vi "1553B_帧解析_字符串_v4.vi"(11 "输入簇":T1) -> (2 "脉冲数":string, 3 "温度":string)   [LabVIEW 2012]
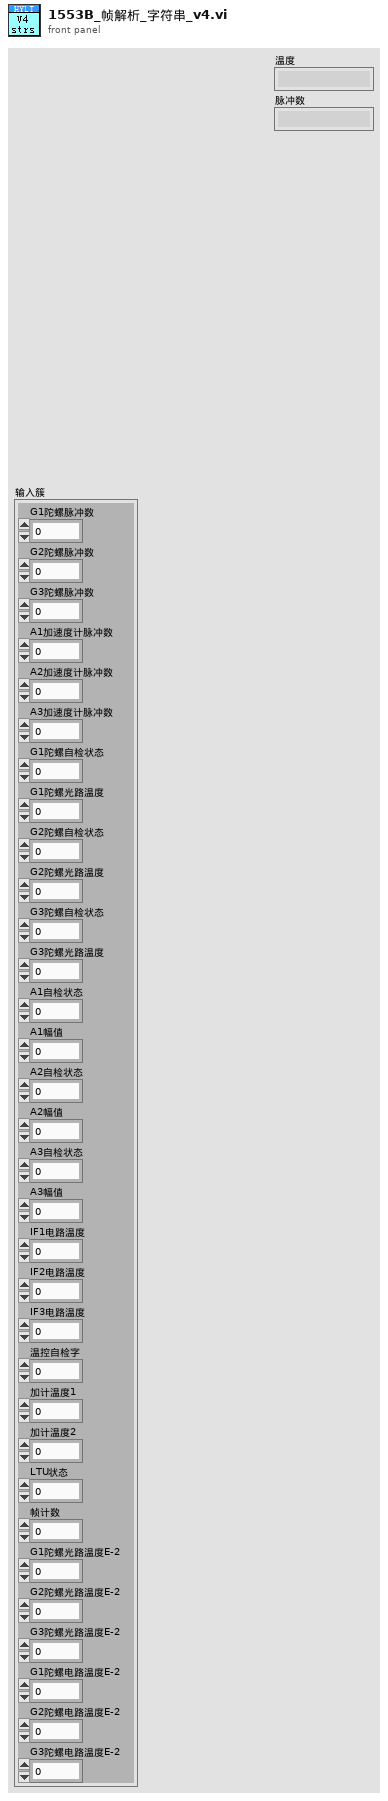
[diagram p1: front panel]
types:
  T1 = cluster{"G1陀螺脉冲数":i32, "G2陀螺脉冲数":i32, "G3陀螺脉冲数":i32, "A1加速度计脉冲数":i16, "A2加速度计脉冲数":i16, "A3加速度计脉冲数":i16, "G1陀螺自检状态":u8, "G1陀螺光路温度":i8, "G2陀螺自检状态":u8, "G2陀螺光路温度":i8, "G3陀螺自检状态":u8, "G3陀螺光路温度":i8, "A1自检状态":u8, "A1幅值":u8, "A2自检状态":u8, "A2幅值":u8, "A3自检状态":u8, "A3幅值":u8, "IF1电路温度":i8, "IF2电路温度":i8, "IF3电路温度":i8, "温控自检字":u8, "加计温度1":i16, "加计温度2":i16, "LTU状态":u8, "帧计数":u8, "G1陀螺光路温度E-2":i16, "G2陀螺光路温度E-2":i16, "G3陀螺光路温度E-2":i16, "G1陀螺电路温度E-2":i16, "G2陀螺电路温度E-2":i16, "G3陀螺电路温度E-2":i16}
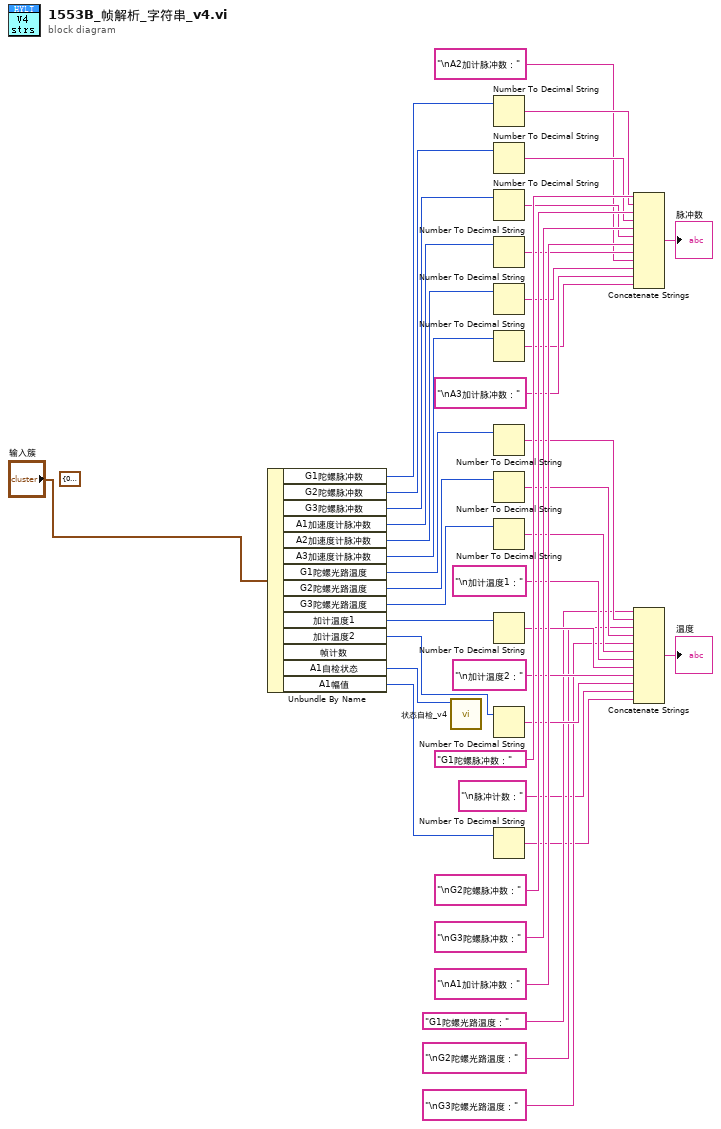
[diagram p0: block diagram]
diagram:
  (unwired) T1 {"G1陀螺脉冲数"=0, "G2陀螺脉冲数"=0, "G3陀螺脉冲数"=0, "A1加速度计脉冲数"=0, "A2加速度计脉冲数"=0, "A3加速度计脉冲数"=0, "G1陀螺自检状态"=0, "G1陀螺光路温度"=0, "G2陀螺自检状态"=0, "G2陀螺光路温度"=0, "G3陀螺自检状态"=0, "G3陀螺光路温度"=0, "A1自检状态"=0, "A1幅值"=0, "A2自检状态"=0, "A2幅值"=0, "A3自检状态"=0, "A3幅值"=0, "IF1电路温度"=0, "IF2电路温度"=0, "IF3电路温度"=0, "温控自检字"=0, "加计温度1"=0, "加计温度2"=0, "LTU状态"=0, "帧计数"=0, "G1陀螺光路温度E-2"=0, "G2陀螺光路温度E-2"=0, "G3陀螺光路温度E-2"=0, "G1陀螺电路温度E-2"=0, "G2陀螺电路温度E-2"=0, "G3陀螺电路温度E-2"=0} ("输入簇")
  n1 = Unbundle By Name("输入簇") -> ("G1陀螺脉冲数"=w25:i32, "G2陀螺脉冲数"=w24:i32, "G3陀螺脉冲数"=w23:i32, "A1加速度计脉冲数"=w22:i16, "A2加速度计脉冲数"=w39:i16, "A3加速度计脉冲数"=w38:i16, "G1陀螺光路温度"=w11:i8, "G2陀螺光路温度"=w10:i8, "G3陀螺光路温度"=w9:i8, "加计温度1"=w8:i16, "加计温度2"=w7:i16, "A1自检状态"=w40:u8, "A1幅值"=w3:u8)  [unwired: 1 out]
  n2 = call "状态自检_v4.vi"("陀螺自检状态字"=w40) -> ()  [unwired: 10 in, 1 out]
  n3 = Number To Decimal String(number=w25) -> (decimal integer string=w36:string)  [unwired: 1 in]
  n4 = Number To Decimal String(number=w24) -> (decimal integer string=w34:string)  [unwired: 1 in]
  n5 = Number To Decimal String(number=w23) -> (decimal integer string=w32:string)  [unwired: 1 in]
  n6 = Number To Decimal String(number=w22) -> (decimal integer string=w30:string)  [unwired: 1 in]
  n7 = Number To Decimal String(number=w39) -> (decimal integer string=w28:string)  [unwired: 1 in]
  n8 = Number To Decimal String(number=w38) -> (decimal integer string=w26:string)  [unwired: 1 in]
  n9 = Number To Decimal String(number=w11) -> (decimal integer string=w13:string)  [unwired: 1 in]
  n10 = Number To Decimal String(number=w10) -> (decimal integer string=w15:string)  [unwired: 1 in]
  n11 = Number To Decimal String(number=w9) -> (decimal integer string=w17:string)  [unwired: 1 in]
  n12 = Number To Decimal String(number=w8) -> (decimal integer string=w19:string)  [unwired: 1 in]
  n13 = Number To Decimal String(number=w7) -> (decimal integer string=w21:string)  [unwired: 1 in]
  n14 = Number To Decimal String(number=w3) -> (decimal integer string=w2:string)  [unwired: 1 in]
  n15 = Concatenate Strings("G1陀螺脉冲数：" ("字符串"), w36, "\nG2陀螺脉冲数：" ("字符串"), w34, "\nG3陀螺脉冲数：" ("字符串"), w32, "\nA1加计脉冲数：" ("字符串"), w30, "\nA2加计脉冲数：" ("字符串"), w28, "\nA3加计脉冲数：" ("字符串"), w26) -> (→"脉冲数":string)
  n16 = Concatenate Strings("G1陀螺光路温度：" ("字符串"), w13, "\nG2陀螺光路温度：" ("字符串"), w15, "\nG3陀螺光路温度：" ("字符串"), w17, "\n加计温度1：" ("字符串"), w19, "\n加计温度2：" ("字符串"), w21, "\n脉冲计数：" ("字符串"), w2) -> (→"温度":string)
